vi "KeyBoardSimulationForTargetVI.vi"(0 "VI Reference In":refnum<vi>, 5 "Control Path":string, 7 "Key Array":T3(array[cluster]) {"Key" items=["LBUTTON"=1, "RBUTTON"=2, "CANCEL"=3, "MBUTTON"=4, "BACKSPACE"=8, "TAB"=9, "CLEAR"=12, "ENTER"=13, "SHIFT"=16, "CTRL"=17, "ALT"=18, "PAUSE"=19, "CAPITAL"=20, "ESCAPE"=27, "SPACE"=32, "PAGEUP"=33, "PAGEDOWN"=34, "END"=35, "HOME"=36, "LEFTARROW"=37, "UPARROW"=38, "RIGHTARROW"=39, "DOWNARROW"=40, "SELECT"=41, "PRINT"=42, "EXECUTE"=43, "PRINTSCREEN"=44, "INSERT"=45, "DELETE"=46, "HELP"=47, "0"=48, "1"=49, "2"=50, "3"=51, "4"=52, "5"=53, "6"=54, "7"=55, "8"=56, "9"=57, "A"=65, "B"=66, "C"=67, "D"=68, "E"=69, "F"=70, "G"=71, "H"=72, "I"=73, "J"=74, "K"=75, "L"=76, "M"=77, "N"=78, "O"=79, "P"=80, "Q"=81, "R"=82, "S"=83, "T"=84, "U"=85, "V"=86, "W"=87, "X"=88, "Y"=89, "Z"=90, "LWIN"=91, "RWIN"=92, "APPS"=93, "NUMPAD0"=96, "NUMPAD1"=97, "NUMPAD2"=98, "NUMPAD3"=99, "NUMPAD4"=100, "NUMPAD5"=101, "NUMPAD6"=102, "NUMPAD7"=103, "NUMPAD8"=104, "NUMPAD9"=105, "MULTIPLY"=106, "ADD"=107, "SEPERATOR"=108, "SUBTRACT"=109, "DECIMAL"=110, "DIVIDE"=111, "F1"=112, "F2"=113, "F3"=114, "F4"=115, "F5"=116, "F6"=117, "F7"=118, "F8"=119, "F9"=120, "F10"=121, "F11"=122, "F12"=123, "F13"=124, "F14"=125, "F15"=126, "F16"=127, "F17"=128, "F18"=129, "F19"=130, "F20"=131, "F21"=132, "F22"=133, "F23"=134, "F24"=135, "NUMLOCK"=144, "SCROLL"=145, "LSHIFT"=160, "RSHIFT"=161, "LCTRL"=162, "RCTRL"=163, "LALT"=164, "RALT"=165, "VOLMUTE"=173, "VOLDOWN"=174, "VOLUP"=175, ";    :"=186, "=   +"=187, ",    <"=188, "-    _"=189, ".    >"=190, "/    ?"=191, "`    ~"=192, "[    {"=219, "\\    |"=220, "]    }"=221, "'    \""=222]}, 11 "error In":errorcluster) -> (4 "VI Reference Out":refnum<vi>, 15 "error IO":errorcluster)   [LabVIEW 2016, in "Drona.lvlib" / "KeyboardSimulation.lvlib"]
doc: "Uses simulated Key Presses to type into a String/Numeric control programmatically. \nThe input control name is given as a string , incase of path, use delimiters inbetween the path."
uses:
  KeyboardSimulation.lvlib
  typedef/VirtualKey.ctl
  typedef/Action.ctl
  Get/GetControlRef/GetControlRefByPath.vi
  Get/GetControlRef/GetControlRef.lvlib
  VI/VI.lvlib
panel:
  # "Overview: This VI is an example that uses simulated Key Presses to type into a control programmatically.  \n\nInstructions:\n1. Enter the keys in the Key Array control. It is what defines which keys are pressed and for how long.  Note that the shift key is pushed down and up in separate steps and that the alphabetical keys are pressed. This is equivalent to holding the shift key down while pressing\n'H', the result being an uppercase 'H'.\n2. Run this VI and 'Hello' will be programmatically typed in the Output box."
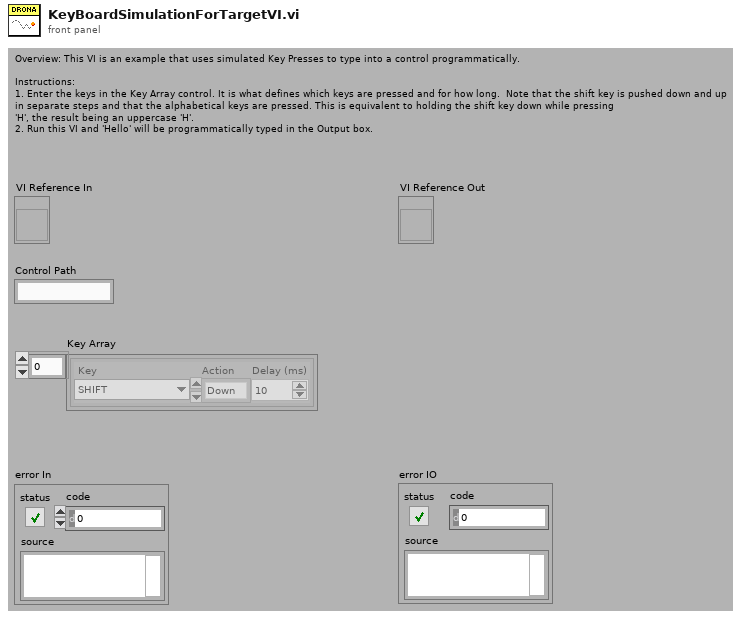
[diagram p1: front panel]
types:
  T1 = typedef "Drona.lvlib/KeyboardSimulation.lvlib/VirtualKey.ctl" = u8
  T2 = typedef "Drona.lvlib/KeyboardSimulation.lvlib/Action.ctl" = enum16{"Press", "Up", "Down"}
  T3 = cluster{" Key":T1, "Action":T2, "Delay (ms)":u32}[]
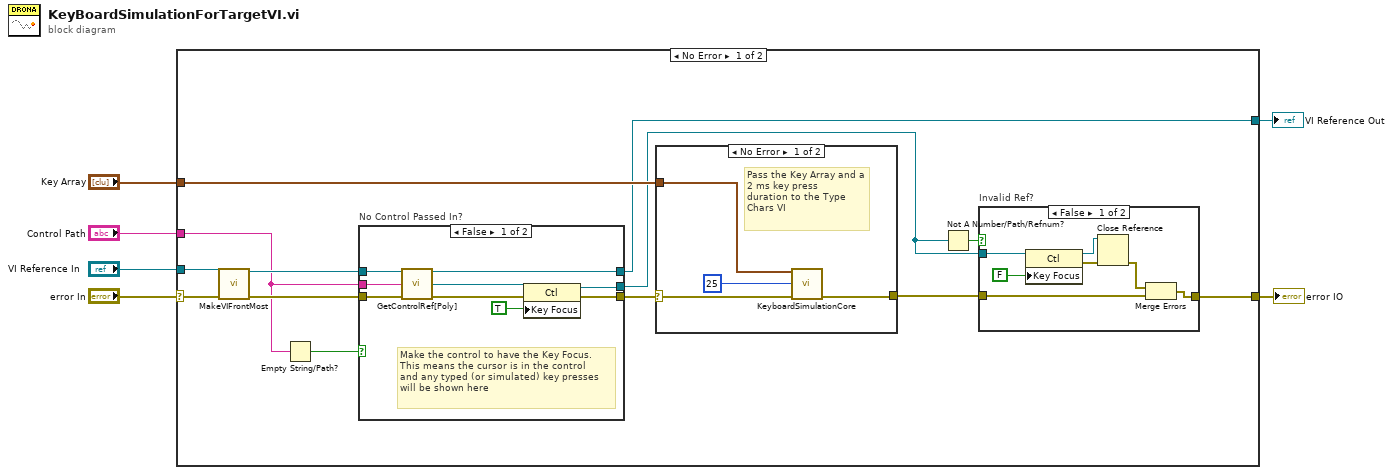
[diagram p0: block diagram]
diagram:
  n1 = case shown="No Error" "error In" {
    selector: "error In" -> [w15 w44]
    tunnel: [w7 w44] -> w6
    tunnel: "Key Array" -> [w18 _]
    tunnel: [w17 w45] -> w4
    tunnel: "VI Reference In" -> [w14 w45]
    tunnel: "Control Path" -> [w12 _]
    frame No Error {
      n2 = call "MakeVIFrontMost.vi"("VI Reference In"=w14, "error in"=w15) -> ("VI Reference Out"=w13:refnum<vi>, "error out"=w16:errorcluster)  [unwired: 12 in]
      n3 = Empty String/Path?(string/path=w12) -> (empty?=w11:bool)
      n4 = case "No Control Passed In?" shown="False" w11 {
        tunnel: [w27 w30] -> w19
        tunnel: [w26 _] -> w9
        tunnel: [w25 w29] -> w17
        tunnel: w16 -> [w22 w30]
        tunnel: w13 -> [w21 w29]
        tunnel: w12 -> [w20 _]
        frame False {
          # "Make the control to have the Key Focus.\nThis means the cursor is in the control\nand any typed (or simulated) key presses\nwill be shown here"
          n5 = call-poly "GetControlRef[Poly].vi"("VI Reference In"=w21, "Control Path"=w20, "error In"=w22) -> ("VI Reference Out"=w25:refnum<vi>, "Ctl Refnum"=w24:refnum<vi>, "error out"=w28:errorcluster)  [unwired: 10 in]
          n6 = property class="Ctl"(reference=w24, error in=w28, "Key Focus"=TRUE) -> (reference out=w26:refnum<vi>, error out=w27:errorcluster)
        }
        frame True {
        }
      }
      n7 = case shown="No Error" w19 {
        selector: w19 -> [w32 w35]
        tunnel: [w31 w35] -> w8
        tunnel: w18 -> [w34 _]
        frame No Error {
          # "Pass the Key Array and a 2 ms key press\nduration to the Type Chars VI"
          n8 = call "KeyboardSimulationCore.vi"("Key Array"=w34, "Length of Key Press (ms)"=u32 25, "error in"=w32) -> ("error out"=w31:errorcluster)  [unwired: 12 in]
        }
        frame Error {
        }
      }
      n9 = Not A Number/Path/Refnum?(number/path/refnum=w9) -> (NaN/Path/Refnum?=w10:bool)
      n10 = case "Invalid Ref?" shown="False" w10 {
        tunnel: [w36 w43] -> w7
        tunnel: w9 -> [w39 _]
        tunnel: w8 -> [w37 w43]
        frame False {
          n11 = property class="Ctl"(reference=w39, "Key Focus"=FALSE) -> (reference out=w40:refnum<vi>, error out=w42:errorcluster)  [unwired: 1 in]
          n12 = Close Reference(reference=w40, error in (no error)=w42) -> (error out=w38:errorcluster)
          n13 = Merge Errors(w38, w37) -> (w36:errorcluster)
        }
        frame True {
        }
      }
    }
    frame Error {
    }
  }
  "error IO" <- w6
  "VI Reference Out" <- w4
